vi "Start Sync.vi"(8 "error in (no error)":errorcluster, 11 "gRPC Server in":refnum<class "TempController_server.lvclass">) -> (0 "error out":errorcluster, 3 "gRPC Server out":refnum<class "TempController_server.lvclass">)   [LabVIEW 2019, in "TempController_server.lvlib" / "TempController_server.lvclass"]
uses:
  TempController_server.lvclass
  TempController_server.lvclass/TempController_server.ctl
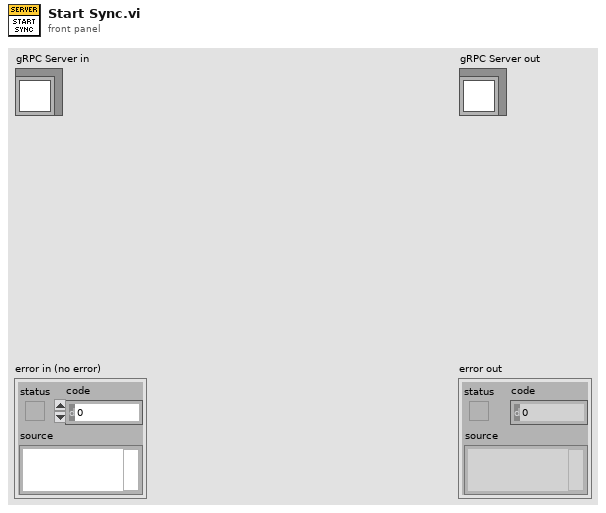
[diagram p1: front panel]
types:
  T1 = typedef "TempController_server.lvlib/TempController_server.lvclass/Server gRPC UEs.ctl" = cluster{"TemperatureControllerService_Measure gRPC UE":refnum<user-event>, "TemperatureControllerService_Configure gRPC UE":refnum<user-event>}
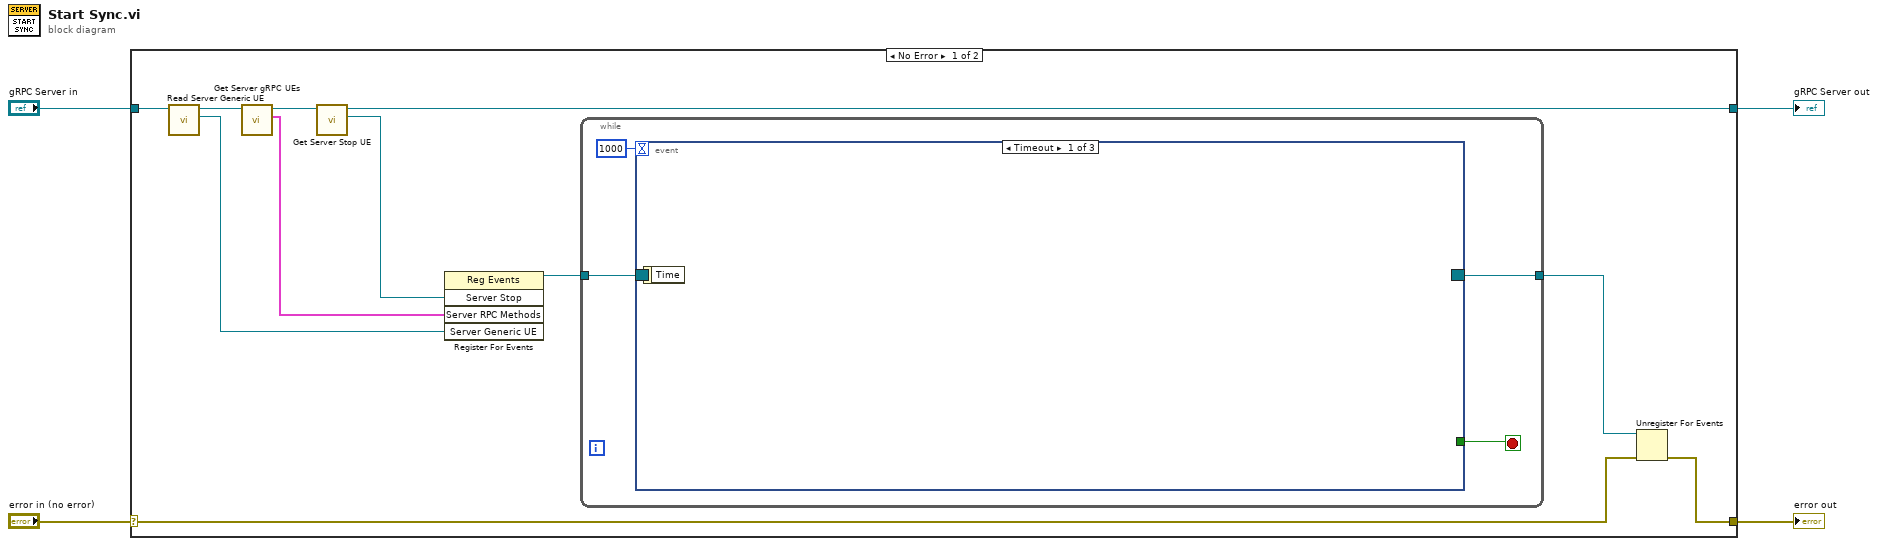
[diagram p0: block diagram]
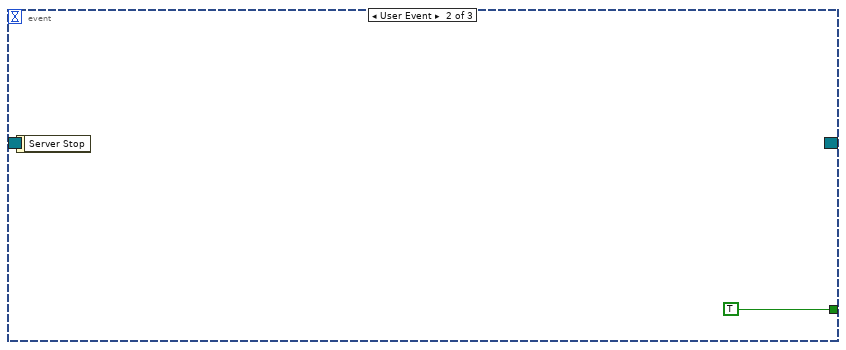
[diagram p2: hidden frame]
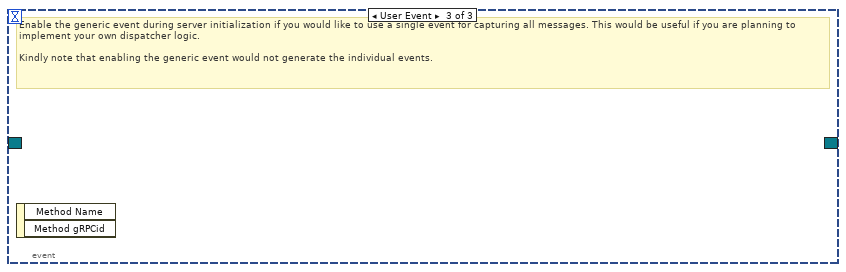
[diagram p3: hidden frame]
diagram:
  n1 = case shown="No Error" "error in (no error)" {
    selector: "error in (no error)" -> [w9 w22]
    tunnel: [w8 w22] -> w3
    tunnel: [w12 w21] -> w1
    tunnel: "gRPC Server in" -> [w7 w21]
    frame No Error {
      n2 = call "Read Server Generic UE.vi"("Template Server in"=w7) -> ("Server Generic UE"=w5:refnum<user-event>, "Template Server out"=w6:refnum<class "TempController_server.lvclass">)  [unwired: 9 in]
      n3 = call "Get Server gRPC UEs.vi"("OOP Server in"=w6) -> ("Server RPC Methods"=w13:T1, "OOP Server out"=w15:refnum<class "TempController_server.lvclass">)  [unwired: 9 in]
      n4 = call "Get Server Stop UE.vi"("OOP Server in"=w15) -> ("Server Stop"=w14:refnum<user-event>, "OOP Server out"=w12:refnum<class "TempController_server.lvclass">)  [unwired: 9 in]
      n5 = register-events(w14, w13, w5) -> (reference out=w11:refnum<event-registration>)  [unwired: 2 in, 1 out]
      n6 = while {
        tunnel: w11 -> [w19]
        tunnel: [w17] -> w10
        stop <- w18 stop-if-true
        n7 = event "RPC Methods Event Structure" shown="[0] Timeout" {
          selector: w19 -> [_ _ _]
          dyn-events: [_ _ _] -> w17
          timeout: 1000 -> [_ _ _]
          tunnel: [_ TRUE _] -> w18
          event Timeout {
            n8 = event-data() -> ()  [unwired: 1 in, 1 out]
          }
          event User Event {
            n9 = event-data() -> ()  [unwired: 1 in, 1 out]
          }
          event User Event {
            # "Enable the generic event during server initialization if you would like to use a single event for capturing all messages. This would be useful if you are planning to implement your own dispatcher logic. \n\nKindly note that enabling the generic event would not generate the individual events."
            n10 = event-data() -> ()  [unwired: 1 in, 2 out]
          }
        }
      }
      n11 = Unregister For Events(event registration refnum=w10, error in=w9) -> (error out=w8:errorcluster)
    }
    frame Error {
    }
  }
  "error out" <- w3
  "gRPC Server out" <- w1
